vi "query control parameters.vi"(8 "error in (no error)":errorcluster, 11 "VISA session":refnum<visa-resource-name>) -> (0 "error out":errorcluster, 1 "Ramp Rate":dbl=3500.0 min=0.0 max=999000.0 step=1e-08 format="%^.5e", 2 "Integral (reset)":dbl=1.0 min=1.0 max=1000.0 step=1e-05 format="%^.5e", 3 "dup VISA session":refnum<visa-resource-name>, 4 "Control Slope Limit":dbl=10.0 min=0.01 max=1000.0 step=1e-05 format="%^.5e", 5 "Proportional (gain)":dbl=10.000000000007324 min=0.01 max=1000.0 step=1e-05 format="%^.5e")   [LabVIEW 2017]
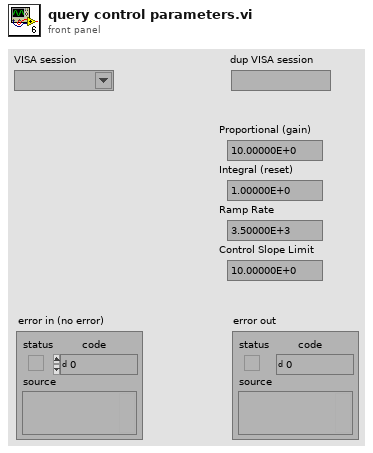
[diagram p1: front panel]
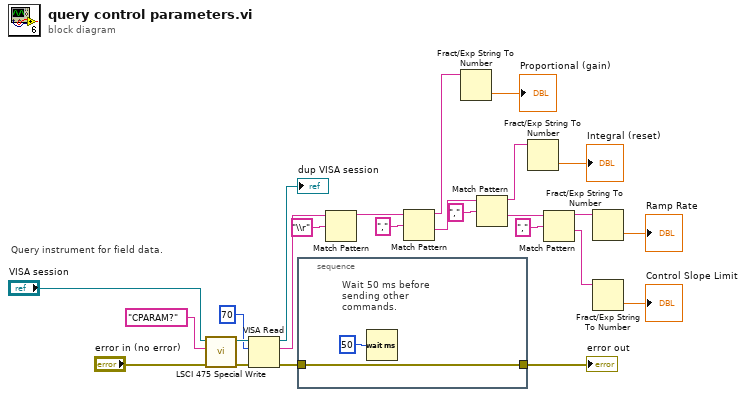
[diagram p0: block diagram]
diagram:
  # "Query instrument for field data."
  n1 = call "LSCI 475 Special Write.vi"("error in (no error)"="error in (no error)", "Write Buffer (\"\")"="CPARAM?", "VISA session"="VISA session") -> ("error out"=w21:errorcluster, "dup VISA session"=w22:refnum<visa-resource-name>)  [unwired: 6 in, 1 out]
  n2 = VISA Read(VISA resource name=w22, byte count=u32 70, error in (no error)=w21) -> (VISA resource name out=→"dup VISA session":refnum<visa-resource-name>, read buffer=w19:string, error out=w16:errorcluster)  [unwired: 1 out]
  n3 = stacked-sequence {
    tunnel: w16 -> [w26]
    tunnel: [w26] -> w15
    frame #0 {
      # "Wait 50 ms before\nsending other\ncommands."
      n4 = Wait (ms)(milliseconds to wait=u32 50) -> ()  [unwired: 1 out]
    }
  }
  "error out" <- w15
  n5 = Match Pattern(string=w19, regular expression="\\r") -> (before substring=w13:string)  [unwired: 1 in, 3 out]
  n6 = Match Pattern(string=w13, regular expression=",") -> (before substring=w8:string, after substring=w11:string)  [unwired: 1 in, 2 out]
  n7 = Fract/Exp String To Number(string=w8) -> (number=→"Proportional (gain)":dbl)  [unwired: 3 in, 1 out]
  n8 = Match Pattern(string=w11, regular expression=",") -> (before substring=w6:string, after substring=w9:string)  [unwired: 1 in, 2 out]
  n9 = Fract/Exp String To Number(string=w6) -> (number=→"Integral (reset)":dbl)  [unwired: 3 in, 1 out]
  n10 = Match Pattern(string=w9, regular expression=",") -> (before substring=w4:string, after substring=w2:string)  [unwired: 1 in, 2 out]
  n11 = Fract/Exp String To Number(string=w4) -> (number=→"Ramp Rate":dbl)  [unwired: 3 in, 1 out]
  n12 = Fract/Exp String To Number(string=w2) -> (number=→"Control Slope Limit":dbl)  [unwired: 3 in, 1 out]
